vi "DistanceToEncoder.vi"(11 "Distance (in)":dbl) -> (3 "Encoder Ticks":dbl)   [LabVIEW 2015]
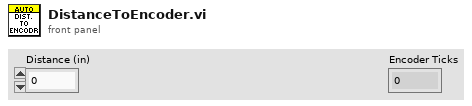
[diagram p1: front panel]
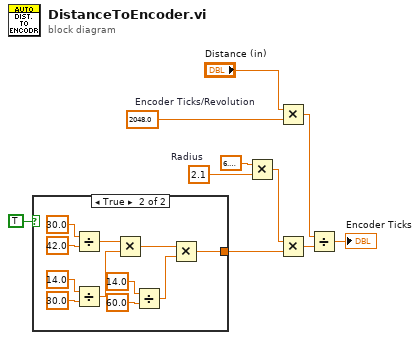
[diagram p0: block diagram]
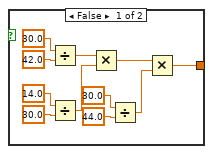
[diagram p2: hidden frame]
diagram:
  w3 = 2.1  # Radius
  w4 = 2048.0  # Encoder Ticks/Revolution
  n1 = case shown="True" TRUE {
    tunnel: [w11 w22] -> w2
    frame False {
      n2 = Divide(x=30.0, y=42.0) -> (x/y=w15:dbl)
      n3 = Divide(x=14.0, y=30.0) -> (x/y=w14:dbl)
      n4 = Multiply(x=w15, y=w14) -> (x*y=w13:dbl)
      n5 = Divide(x=30.0, y=44.0) -> (x/y=w12:dbl)
      n6 = Multiply(x=w13, y=w12) -> (x*y=w11:dbl)
    }
    frame True {
      n7 = Divide(x=30.0, y=42.0) -> (x/y=w26:dbl)
      n8 = Divide(x=14.0, y=30.0) -> (x/y=w25:dbl)
      n9 = Multiply(x=w26, y=w25) -> (x*y=w24:dbl)
      n10 = Divide(x=14.0, y=60.0) -> (x/y=w23:dbl)
      n11 = Multiply(x=w24, y=w23) -> (x*y=w22:dbl)
    }
  }
  n12 = Multiply(x=6.283185307179586, y=w3) -> (x*y=w5:dbl)
  n13 = Multiply(x="Distance (in)", y=w4) -> (x*y=w9:dbl)
  n14 = Multiply(x=w5, y=w2) -> (x*y=w8:dbl)
  n15 = Divide(x=w9, y=w8) -> (x/y=→"Encoder Ticks":dbl)
